vi "WFRepetitionsNULL.vi"() -> (3 "Repetitions":T1 {"Interval (s)" min=0.0; "Delay (s)" min=0.0})   [LabVIEW 2009]
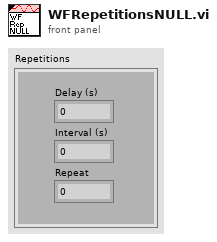
[diagram p1: front panel]
types:
  T1 = cluster{"Delay (s)":dbl, "Interval (s)":dbl, "Repeat":i32}
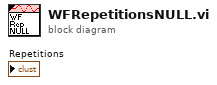
[diagram p0: block diagram]
diagram:
